vi "20151006_HW3_0412107_陳麒升.vi"() -> ()   [LabVIEW 2014]
panel:
  out "正確率":i16
  out "sum":i16
  out "abs(x)":i16[][](array[numeric])
  out "String":string
  out "0, 2":i16[][](array[numeric])
  out "0, 1":i16[][](array[numeric])
  in  "等級(1~10)":i32=3
  in  "?":bool
  out "剩餘秒數":u32
  in  "挑戰區":bool[][](array[boolean])
  out "關卡區":bool[][](array[boolean])
  # "跑馬燈記憶"
  # "(傳說級)"
  # "說明：請先選擇關卡等級後按下執行後關卡區會隨機出現一\n           組LED的排列組合，您有20秒的時間去快速記憶此組合\n           並於20秒後於挑戰區按出您剛記憶的組合，挑戰完點擊\n           \"完成\"鍵將按正確比例計分(滿分100)並輸出等級(最高為\n           S rank)。"
  # "背景圖片來源為www.popd.hk"
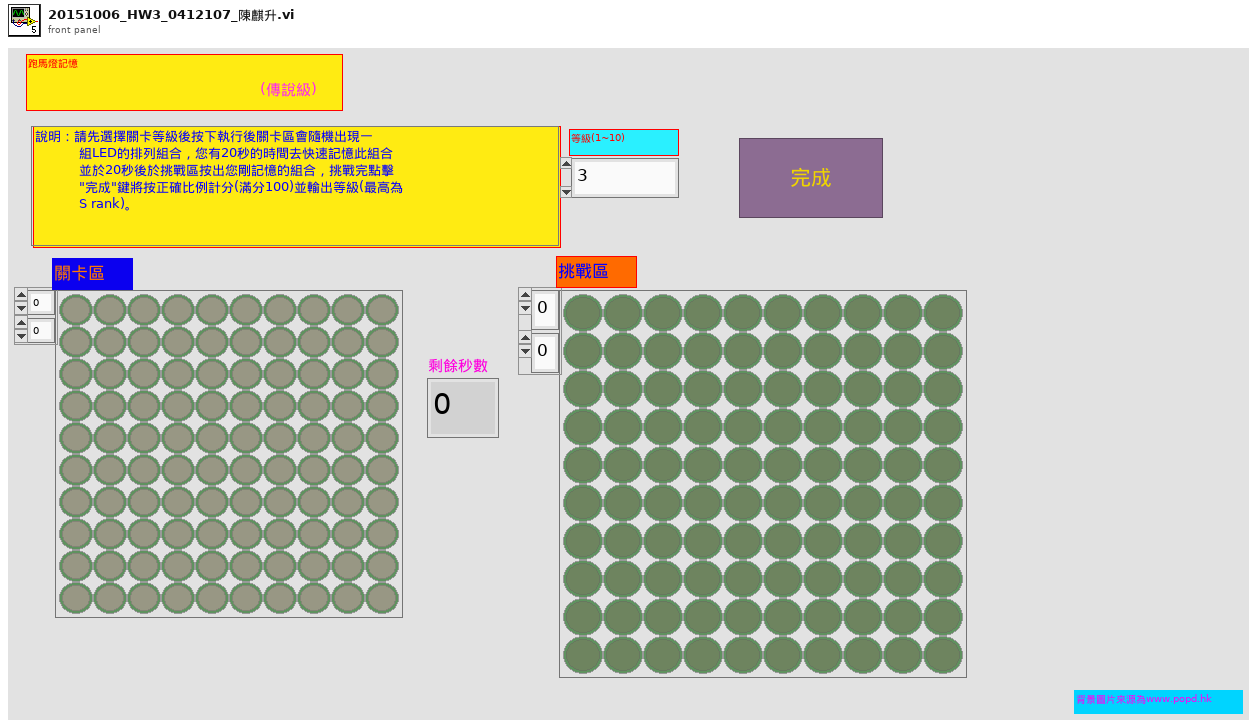
[diagram p1: front panel]
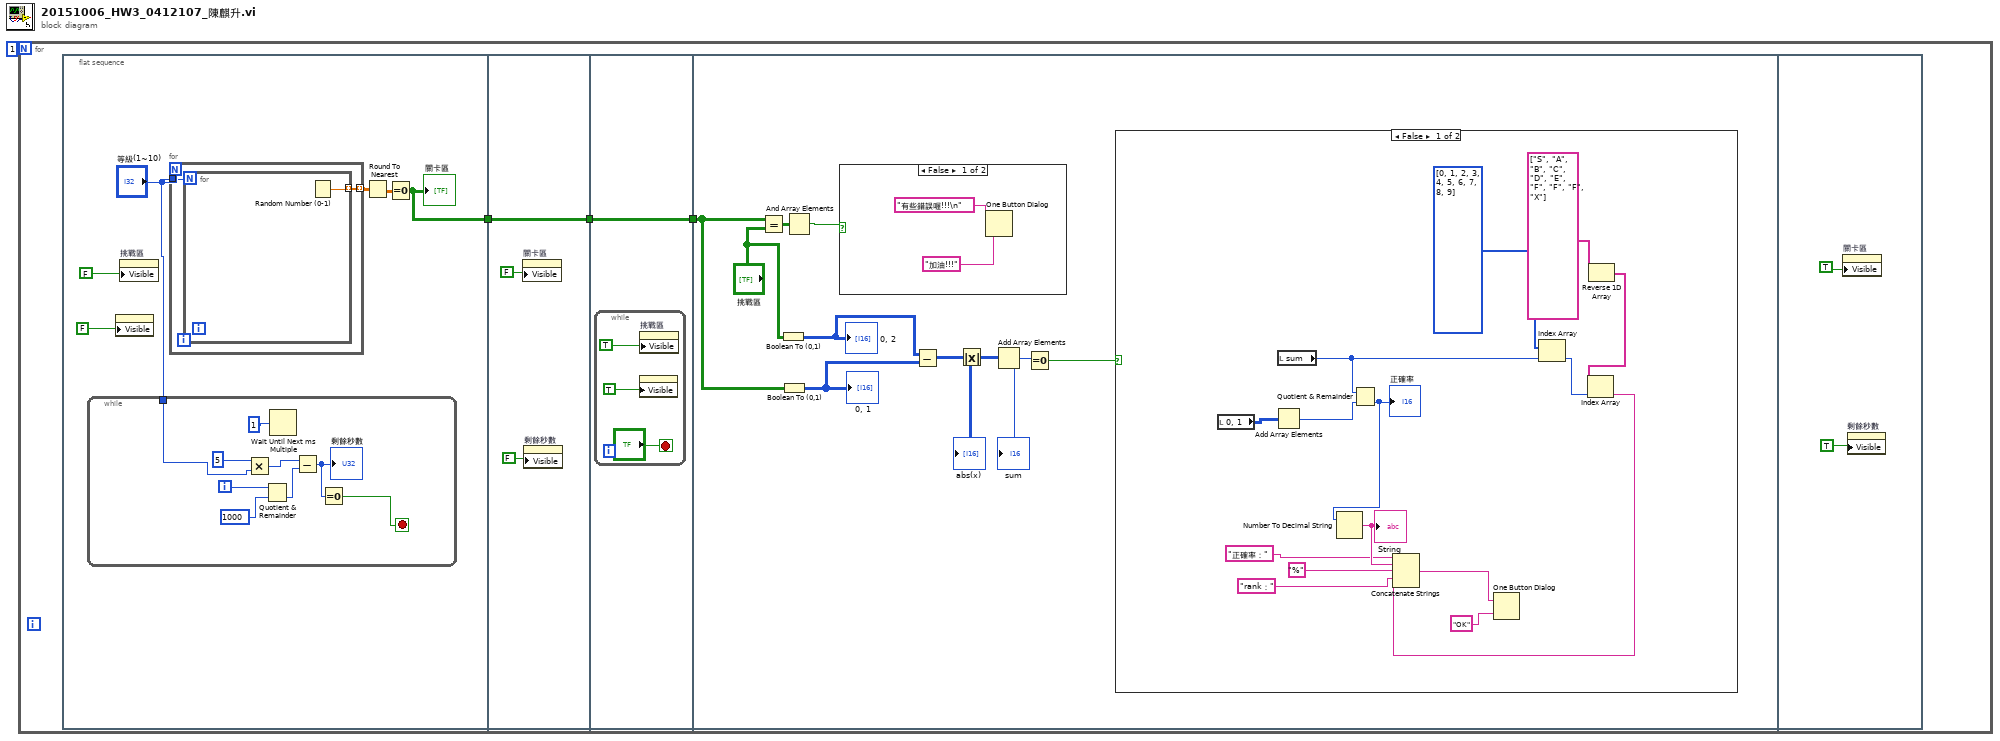
[diagram p0: block diagram]
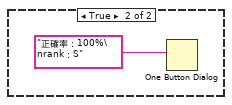
[diagram p2: hidden frame]
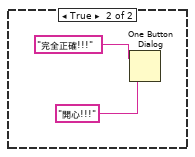
[diagram p3: hidden frame]
diagram:
  n1 = for {
    N: 1 -> [_]
    n2 = flat-sequence {
      tunnel: [w7] -> w4
      tunnel: w4 -> [w23]
      tunnel: [w23] -> w3
      tunnel: w3 -> [w26]
      tunnel: [w26] -> w2
      tunnel: w2 -> [w37]
      frame #0 {
        n3 = while {
          tunnel: "等級(1~10)" -> [w12]
          i -> [w17]
          stop <- w11 stop-if-true
          n4 = Multiply(x=5, y=w12) -> (x*y=w13:i32)
          n5 = Quotient & Remainder(x=w17, y=1000) -> (floor(x/y)=w15:i32)  [unwired: 1 out]
          n6 = Wait Until Next ms Multiple(millisecond multiple=u32 1) -> ()  [unwired: 1 out]
          n7 = Subtract(x=w13, y=w15) -> (x-y=w18:i32)
          "剩餘秒數" <- w18
          n8 = Equal To 0?(x=w18) -> (x = 0?=w11:bool)
        }
        n9 = property class="Bool"("Visible"=FALSE) -> ()  [unwired: 2 in, 2 out]
        n10 = property on="挑戰區" class="Arr (strict)"("Visible"=FALSE) -> ()  [unwired: 2 in, 2 out]
        n11 = for {
          N: "等級(1~10)" -> [_]
          tunnel: [w21] -> w10 mode=indexing
          tunnel: "等級(1~10)" -> [w20]
          n12 = for {
            N: w20 -> [_]
            tunnel: [w22] -> w21 mode=indexing
            n13 = Random Number (0-1)() -> (number: 0 to 1=w22:dbl)
          }
        }
        n14 = Round To Nearest(number=w10) -> (nearest integer value=w9:dbl[][])
        n15 = Equal To 0?(x=w9) -> (x = 0?=w7:bool[][])
        "關卡區" <- w7
      }
      frame #1 {
        n16 = property on="關卡區" class="Arr (strict)"("Visible"=FALSE) -> ()  [unwired: 2 in, 2 out]
        n17 = property on="剩餘秒數" class="DigNum (strict)"("Visible"=FALSE) -> ()  [unwired: 2 in, 2 out]
      }
      frame #2 {
        n18 = while {
          stop <- "?" stop-if-true
          n19 = property class="Bool"("Visible"=TRUE) -> ()  [unwired: 2 in, 2 out]
          n20 = property on="挑戰區" class="Arr (strict)"("Visible"=TRUE) -> ()  [unwired: 2 in, 2 out]
        }
      }
      frame #3 {
        n21 = Equal?(x=w37, y="挑戰區") -> (x = y?=w39:bool[][])
        n22 = Boolean To (0,1)(Boolean="挑戰區") -> (0, 1=w35:i16[][])
        "0, 2" <- w35
        n23 = Boolean To (0,1)(Boolean=w37) -> (0, 1=w34:i16[][])
        "0, 1" <- w34
        n24 = And Array Elements(Boolean array=w39) -> (logical AND=w38:bool)
        n25 = case shown="False" w38 {
          frame False {
            n26 = One Button Dialog(message="有些錯誤喔!!!\n", button name ("OK")="加油!!!") -> ()  [unwired: 1 out]
          }
          frame True {
            n27 = One Button Dialog(message="完全正確!!!", button name ("OK")="開心!!!") -> ()  [unwired: 1 out]
          }
        }
        n28 = Subtract(x=w35, y=w34) -> (x-y=w33:i16[][])
        n29 = Absolute Value(x=w33) -> (abs(x)=w32:i16[][])
        "abs(x)" <- w32
        n30 = Add Array Elements(numeric array=w32) -> (sum=w31:i16)
        "sum" <- w31
        n31 = Equal To 0?(x=w31) -> (x = 0?=w30:bool)
        n32 = case shown="False" w30 {
          frame False {
            n33 = local read "0, 1"() -> (w45:i16[][])
            n34 = Add Array Elements(numeric array=w45) -> (sum=w43:i16)
            n35 = local read "sum"() -> (w44:i16)
            n36 = Quotient & Remainder(x=w44, y=w43) -> (floor(x/y)=w42:i16)  [unwired: 1 out]
            "正確率" <- w42
            n37 = Number To Decimal String(number=w42) -> (decimal integer string=w48:string)  [unwired: 1 in]
            "String" <- w48
            n38 = Index Array(array=i32[] [0, 1, 2, 3, 4, 5, 6, 7, 8, 9] ("Array 2"), index=w44) -> (element=w51:i32)
            n39 = Reverse 1D Array(array=string[] ["S", "A", "B", "C", "D", "E", "F", "F", "F", "X"] ("Array 3")) -> (reversed array=w53:string[])
            n40 = Index Array(array=w53, index=w51) -> (element=w54:string)
            n41 = Concatenate Strings("正確率：", w48, "%", "rank：" ("string"), w54) -> (w49:string)
            n42 = One Button Dialog(message=w49, button name ("OK")="OK") -> ()  [unwired: 1 out]
          }
          frame True {
            n43 = One Button Dialog(message="正確率：100%\nrank：S") -> ()  [unwired: 1 in, 1 out]
          }
        }
      }
      frame #4 {
        n44 = property on="關卡區" class="Arr (strict)"("Visible"=TRUE) -> ()  [unwired: 2 in, 2 out]
        n45 = property on="剩餘秒數" class="DigNum (strict)"("Visible"=TRUE) -> ()  [unwired: 2 in, 2 out]
      }
    }
  }
